vi "Write Actors to Nest.vi"(10 "Actors to Nest":refnum<class "Actor.lvclass">[](array[class]), 11 "Template in":refnum<class "Template.lvclass">) -> (3 "Template out":refnum<class "Template.lvclass">)   [LabVIEW 2020, in "Template.lvlib" / "Template.lvclass"]
doc: "Sets the channel actors to nest"
uses:
  Template.lvclass
  <vilib>/ActorFramework/Actor/Actor.lvclass
  Template.lvclass/Template.ctl
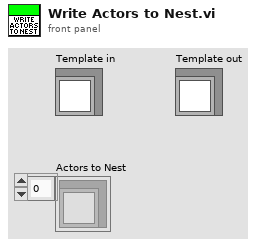
[diagram p1: front panel]
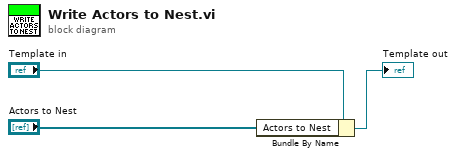
[diagram p0: block diagram]
diagram:
  n1 = Bundle By Name(cluster="Template in", "Actors to Nest"="Actors to Nest") -> (→"Template out":refnum<class "Template.lvclass">)
